vi "Write refOfLvLib.vi"(8 "error in (no error)":errorcluster, 10 "refOfLvLib":refnum<vi>, 11 "LibReader in":refnum<class "LibReader.lvclass">) -> (0 "error out":errorcluster, 3 "LibReader out":refnum<class "LibReader.lvclass">)   [LabVIEW 2018, in "LibReader.lvclass"]
doc: "Write the refrence of LabVIEW library."
uses:
  LibReader.lvclass
  LibReader.lvclass/LibReader.ctl
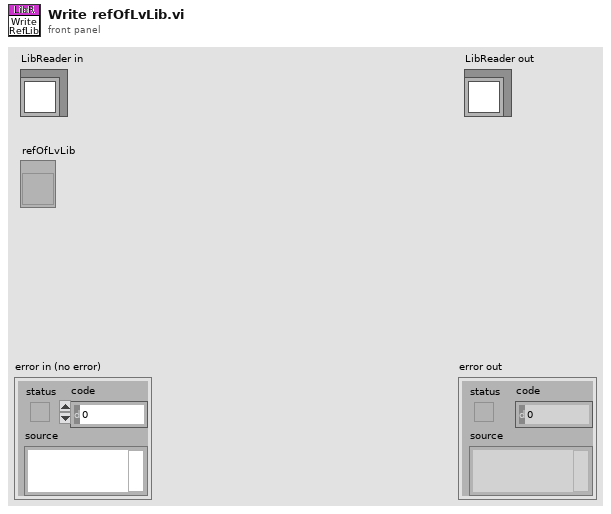
[diagram p1: front panel]
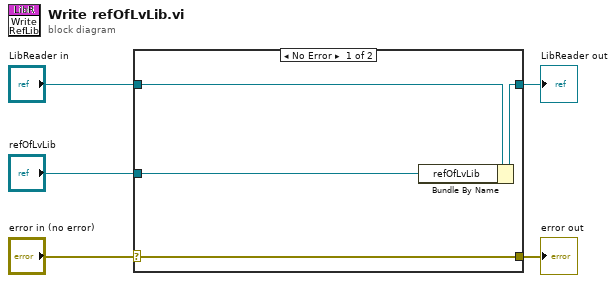
[diagram p0: block diagram]
diagram:
  n1 = case shown="No Error" "error in (no error)" {
    selector: "error in (no error)" -> [w9 w10]
    tunnel: [w9 w10] -> w4
    tunnel: [w7 w11] -> w2
    tunnel: "LibReader in" -> [w8 w11]
    tunnel: "refOfLvLib" -> [w6 _]
    frame No Error {
      n2 = Bundle By Name(cluster=w8, "refOfLvLib"=w6) -> (w7:refnum<class "LibReader.lvclass">)
    }
    frame Error {
    }
  }
  "error out" <- w4
  "LibReader out" <- w2
